vi "setUp.vi"(8 "error in (no error)":errorcluster, 11 "reference in":refnum<class "LVLIBP CD XML Updater Unit Tests.lvclass">) -> (0 "error out":errorcluster, 3 "reference out":refnum<class "LVLIBP CD XML Updater Unit Tests.lvclass">)   [LabVIEW 2018, in "LVLIBP CD XML Updater Unit Tests.lvclass"]
uses:
  LVLIBP CD XML Updater Unit Tests.lvclass
  C:/Program Files (x86)/National Instruments/LabVIEW 2018/vi.lib/addons/_JKI Toolkits/VI Tester/TestCase.llb/TestCase.lvclass
  LVLIBP CD XML Updater Unit Tests.lvclass/LVLIBP CD XML Updater Unit Tests.ctl
  <vilib>/addons/_JKI Toolkits/VI Tester/TestCase.llb/TestCase.lvclass
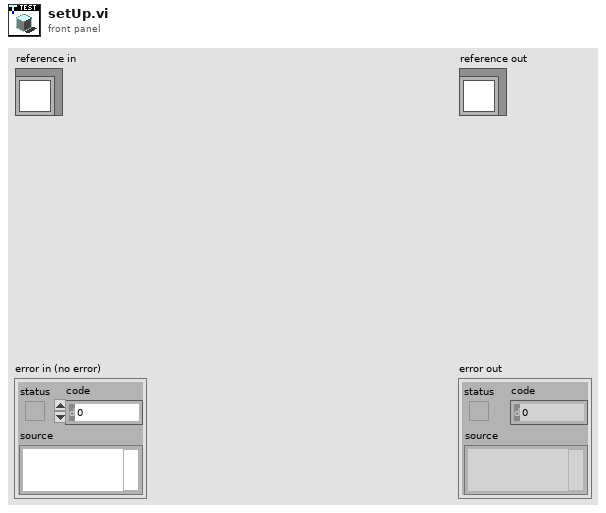
[diagram p1: front panel]
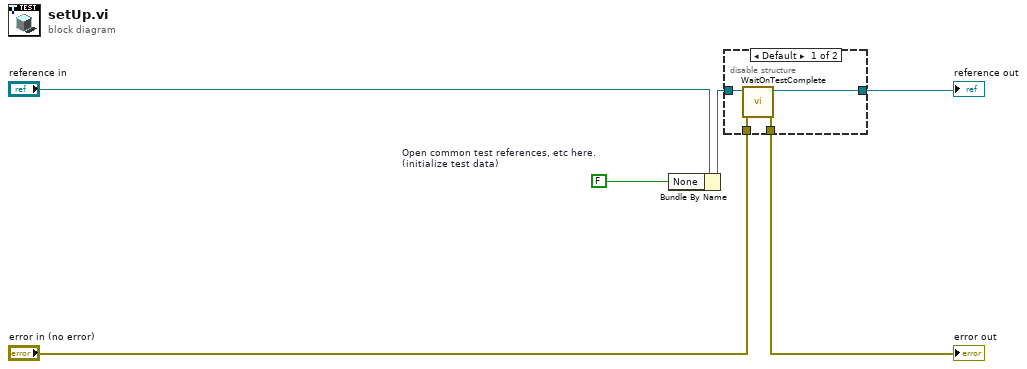
[diagram p0: block diagram]
diagram:
  w5 = FALSE  # Open common test references, etc here. (initialize test data)
  n1 = Bundle By Name(cluster="reference in", "None"=w5) -> (w6:refnum<class "LVLIBP CD XML Updater Unit Tests.lvclass">)
  n2 = disable-structure shown="Default" {
    disable-tunnel: "error in (no error)" -> [w10 w11]
    disable-tunnel: [w9 w11] -> w1
    disable-tunnel: [w8 w12] -> w3
    disable-tunnel: w6 -> [w7 w12]
    frame condition #0 (active) {
      n3 = call <vilib>:"WaitOnTestComplete.vi"("error in (no error)"=w10, "TestCase in"=w7) -> ("error out"=w9:errorcluster, "TestCase out"=w8:refnum<class "LVLIBP CD XML Updater Unit Tests.lvclass">)  [unwired: 8 in]
    }
    frame condition #1 {
    }
  }
  "error out" <- w1
  "reference out" <- w3
